vi "ASIO_Input_Output.vi"() -> ()   [LabVIEW 2016]
uses:
  WaveIO.llb/ASIO_Informations.ctl
  <vilib>/measure/NI_MABase.lvlib
panel:
  out "ASIO Device Infos":T1[](array[typedef])
  out "error rec":errorcluster
  out "Input Data":i32[][](graph)
  out "Rec Error":errorcluster
  out "bufferTime":dbl=16625.487 format="%#.1f"
  out "About":string="WaveIO DLL Version 1.01 (c) C. Zeitnitz 25. August 2014 - with ASIO support"
  in  "card #":u32
  in  "Frequencies":dbl[](array[numeric])=[101.0, 300.0, 500.0, 700.0, 900.0, 1100.0]
  out "Number of Devices":i32=1
  out "Play Error":errorcluster
  in  "Format":cluster{"Rate":i32, "Bits":i32, "Channels":u32}={"Rate"=44100, "Bits"=32, "Channels"=2}
  in  "Buffer":T2={"# buffers"=4, "Buffer size"=2048, "unit (ms)"=enum."Samples"}
  out "error play":errorcluster
  out "Output Data":i32[][](graph)
  in  "Stop":bool=TRUE
  # "JUST FOR INFORMATION\nHas no effect in the code!!"
  # "ONLY FOR ASIO INPUT AND OUTPUT"
  # "ASIO is a trademark and software of Steinberg Media Technologies GmbH"
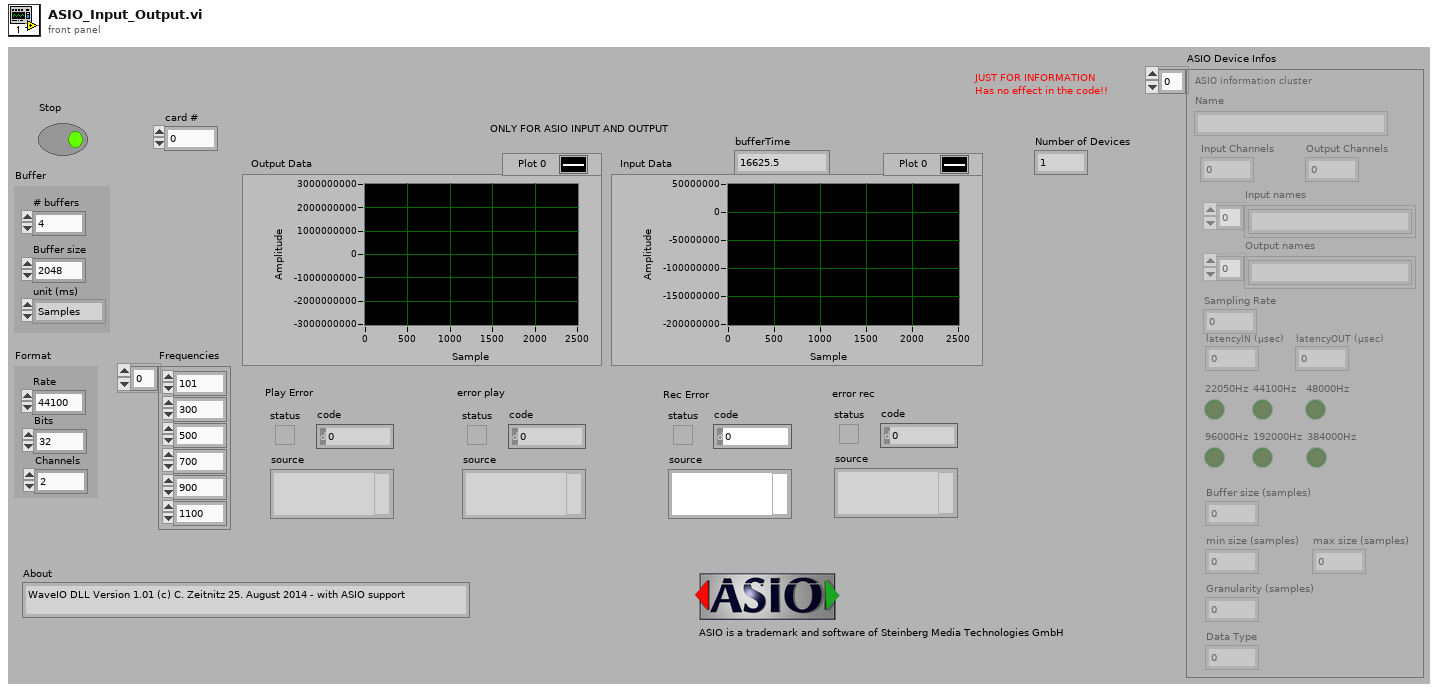
[diagram p1: front panel]
types:
  T1 = typedef "ASIO_Informations.ctl" = cluster{"Input Channels":i32, "Output Channels":i32, "Sampling Rate":i32, "22050Hz":bool, "44100Hz":bool, "48000Hz":bool, "96000Hz":bool, "192000Hz":bool, "Buffer size (samples)":i32, "min size (samples)":i32, "max size (samples)":i32, "Granularity (samples)":i32, "Name":string, "Data Type":i32, "latencyIN (µsec)":i32, "latencyOUT (µsec)":i32, "Input names":string[], "Output names":string[], "384000Hz":bool}
  T2 = cluster{"# buffers":i32, "Buffer size":i32, "unit (ms)":enum16{"time (ms)", "Samples"}}
  T3 = enum16{"Sine Wave", "Triangle Wave", "Square Wave", "Sawtooth Wave"}
  T4 = typedef "SoundHandle.ctl" = cluster{"DeviceID":u16, "Samples/buf":u32, "Sampl rate":u32, "Bits/sample":u16, "Channels":u8, "Opened":bool}
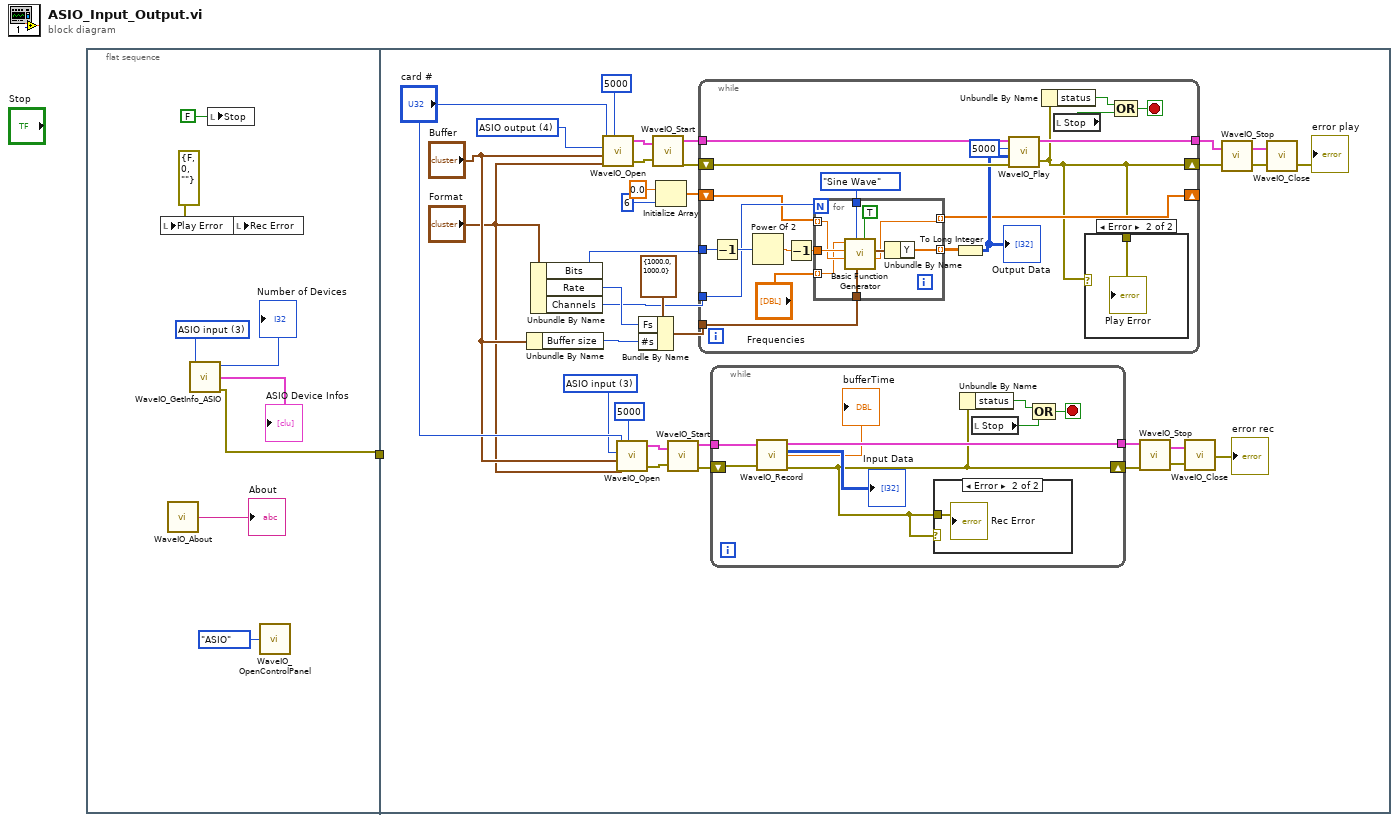
[diagram p0: block diagram]
diagram:
  n1 = flat-sequence {
    tunnel: [w2] -> w1
    tunnel: w1 -> [_]
    frame #0 {
      w6 = u16 3 items=["Input", "Output", "Loopback", "ASIO input", "ASIO output"] ("Direction (Input)")
      w5 = errorcluster {"status"=FALSE, "code"=0, "source"=""} ("Play Error")
      n2 = local write "Play Error"(w5) -> ()
      n3 = call "WaveIO_About.vi"() -> ("About"=→"About":string)  [unwired: 1 in]
      n4 = call "WaveIO_GetInfo_ASIO.vi"("Direction (Input)"=w6) -> ("error out"=w2:errorcluster, "numdev"=→"Number of Devices":i32, "ASIO Device Infos"=→"ASIO Device Infos":T1[])  [unwired: 2 out]
      n5 = local write "Stop"(FALSE ("Stop")) -> ()
      n6 = local write "Rec Error"(w5) -> ()
      n7 = call "WaveIO_OpenControlPanel.vi"("Sound Option"=enum16{"Record", "Playback", "ASIO"}."ASIO") -> ()  [unwired: 1 in]
    }
    frame #1 {
      w10 = u16 4 items=["Record", "Play", "Loopback", "ASIO input", "ASIO output"] ("Direction (Record)")
      w11 = u16 3 items=["Record", "Play", "Loopback", "ASIO input", "ASIO output"] ("Direction (Record)")
      n8 = Unbundle By Name("Buffer") -> ("Buffer size"=w31:i32)
      n9 = Unbundle By Name("Format") -> ("Bits"=w30:i32, "Rate"=w32:i32, "Channels"=w26:u32)
      n10 = call "WaveIO_Open.vi"("idev"="card #", "Watchdog timeout (msec) (default=OFF)"=5000, "device type (Record)"=w10, "Buffer Config"="Buffer", "Format (44kHz, 16Bit, stereo)"="Format") -> ("Sound Handle Out"=w36:T4, "error out"=w35:errorcluster)  [unwired: 2 in]
      n11 = call "WaveIO_Open.vi"("idev"="card #", "Watchdog timeout (msec) (default=OFF)"=5000, "device type (Record)"=w11, "Buffer Config"="Buffer", "Format (44kHz, 16Bit, stereo)"="Format") -> ("Sound Handle Out"=w19:T4, "error out"=w18:errorcluster)  [unwired: 2 in]
      n12 = Bundle By Name(cluster=cluster{"Fs":dbl, "#s":dbl} {"Fs"=1000.0, "#s"=1000.0} ("sampling info"), "Fs"=w32, "#s"=w31) -> (w39:cluster{"Fs":dbl, "#s":dbl})
      n13 = call "WaveIO_Start.vi"("error in (no error)"=w35, "Handle"=w36) -> ("error out"=w37:errorcluster, "Handle Out"=w38:T4)
      n14 = Initialize Array(0.0 ("element"), 6 ("dimension size")) -> (w29:dbl[])
      n15 = call "WaveIO_Start.vi"("error in (no error)"=w18, "Handle"=w19) -> ("error out"=w16:errorcluster, "Handle Out"=w17:T4)
      n16 = while {
        shift-right: [w55] -> w34
        shift-left: w37 -> [w70]
        tunnel: w38 -> [w71]
        tunnel: [w67] -> w42
        tunnel: w39 -> [w68]
        tunnel: w30 -> [w65]
        shift-right: [w57] -> _
        shift-left: w29 -> [w58]
        tunnel: w26 -> [w59]
        stop <- w73 stop-if-true
        n17 = Decrement(x=w65) -> (x-1=w63:i32)
        n18 = Power Of 2(x=w63) -> (2^x=w64:dbl)
        n19 = Decrement(x=w64) -> (x-1=w62:dbl)
        n20 = for {
          N: w59 -> [_]
          tunnel: w68 -> [w81]
          tunnel: T3."Sine Wave" ("signal type") -> [w80]
          tunnel: w62 -> [w79]
          tunnel: [w78] -> w61 mode=indexing
          tunnel: w58 -> [w77] mode=indexing
          tunnel: [w76] -> w57 mode=indexing
          tunnel: "Frequencies" -> [w74] mode=indexing
          n21 = call <vilib>:"Basic Function Generator.vi"("reset signal"=TRUE, "sampling info"=w81, "signal type"=w80, "phase"=w77, "amplitude"=w79, "frequency"=w74) -> ("phase out"=w76:dbl, "signal out"=w82:waveform(dbl))  [unwired: 3 in, 1 out]
          n22 = Unbundle By Name(w82) -> ("Y"=w78:dbl[])
        }
        n23 = To Long Integer(number=w61) -> (32bit integer=w60:i32[][])
        "Output Data" <- w60
        n24 = call "WaveIO_Play.vi"("error in (no error)"=w70, "data"=w60, "timeout (automatic)"=5000, "Handle"=w71) -> ("error out"=w55:errorcluster, "Handle Out"=w67:T4)
        n25 = Unbundle By Name(w55) -> ("status"=w72:bool)
        n26 = local read "Stop"() -> (w69:bool)
        n27 = case shown="Error" w55 {
          tunnel: w55 -> [_ w83]
          frame No Error {
          }
          frame Error {
            "Play Error" <- w83
          }
        }
        n28 = Compound Arithmetic op=OR(w72, w69) -> (w73:bool)
      }
      n29 = while {
        shift-right: [w46] -> w21
        shift-left: w16 -> [w49]
        tunnel: w17 -> [w50]
        tunnel: [w47] -> w23
        stop <- w52 stop-if-true
        n30 = call "WaveIO_Record.vi"("Handle"=w50, "error in (no error)"=w49) -> ("Handle Out"=w47:T4, "Data"=→"Input Data":i32[][], "error out"=w46:errorcluster, "bufferTime [µs]"=→"bufferTime":dbl)  [unwired: 1 in, 1 out]
        n31 = case shown="Error" w46 {
          tunnel: w46 -> [_ w53]
          frame No Error {
          }
          frame Error {
            "Rec Error" <- w53
          }
        }
        n32 = Unbundle By Name(w46) -> ("status"=w51:bool)
        n33 = local read "Stop"() -> (w44:bool)
        n34 = Compound Arithmetic op=OR(w51, w44) -> (w52:bool)
      }
      n35 = call "WaveIO_Stop.vi"("error in (no error)"=w21, "Handle"=w23) -> ("error out"=w22:errorcluster, "Handle Out"=w24:T4)
      n36 = call "WaveIO_Close.vi"("error in (no error)"=w22, "Handle"=w24) -> ("error out"=→"error rec":errorcluster)  [unwired: 1 out]
      n37 = call "WaveIO_Stop.vi"("error in (no error)"=w34, "Handle"=w42) -> ("error out"=w41:errorcluster, "Handle Out"=w43:T4)
      n38 = call "WaveIO_Close.vi"("error in (no error)"=w41, "Handle"=w43) -> ("error out"=→"error play":errorcluster)  [unwired: 1 out]
    }
  }
